vi "NI-DCPower Source DC Voltage.vi"() -> ()   [LabVIEW 2021]
doc: "Demonstrates how to use the DC Voltage Output Function to force an output voltage. This example initializes a session, configures the Output Function, Sense, Autorange, Voltage Level and Current Limit, initiates generation, waits for a specified delay, and measures the voltage and current output. This example uses Single Point source mode."
uses:
  <instrlib>/niDCPower/nidcpower.llb/niDCPower Source Mode.ctl
  <instrlib>/niDCPower/nidcpower.llb/niDCPower Wait For Event - Event.ctl
  <instrlib>/niDCPower/nidcpower.llb/niDCPower Output Function.ctl
  <instrlib>/niDigital/niDigital.llb/niDigital Selected Function.ctl
  <instrlib>/niDigital/niDigital.llb/niDigital Burst Pattern (Pass Fail).vi
  <instrlib>/niDigital/niDigital.llb/niDigital Get Site Results Site Numbers.vi
panel:
  out "Pass?":bool[](array[boolean])
  out "Site":string[](array[string])
  in  "Digital":refnum<k15>="PXI1Slot2,PXI1Slot3" caption="resource name"
  in  "error in":errorcluster
  out "error out":errorcluster
  in  "Source Delay (Sec)":dbl=0.1 format="%.3p"
  out "Voltage Measurement":dbl
  out "Current Measurement":dbl
  in  "Current Limit Range":dbl=0.01 format="%.3p"
  in  "Voltage Level Range":dbl=6.0 format="%.5p"
  in  "Current Limit":dbl=0.01 format="%.3p"
  in  "Voltage Level":dbl=2.0 format="%.5p"
  in  "Vin SMU Channel":string="0"
  in  "Vin SMU":refnum<k15>="Dev1"
  # "Overview: Demonstrates how to use the DC Voltage Output Function to force an output voltage.  \nThis example initializes a session; configures the Output Function, Voltage Level and Current Limit; \ninitiates generation; waits for a specified delay; and measures the voltage and current output. \nRequirements: NI-DCPower\nInstructions:\n1. Select the appropriate device in the Resource Name control.\n2. Configure the parameters of the DC Voltage signal you'd like to output.\n3. Run the VI."
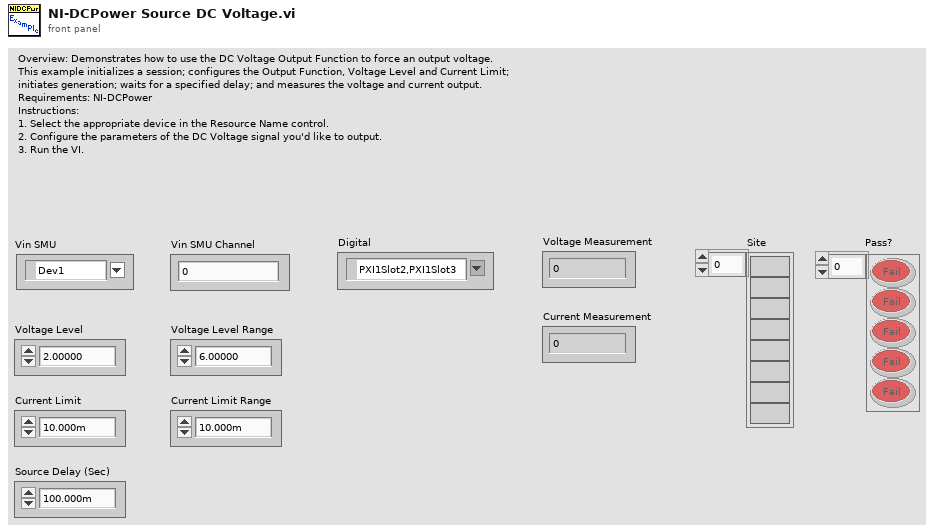
[diagram p1: front panel]
types:
  T1 = typedef "niDigital Selected Function.ctl" = i32
  T2 = typedef "niDCPower Output Function.ctl" = i32
  T3 = typedef "niDCPower Wait For Event - Event.ctl" = i32
  T4 = typedef "niDCPower Source Mode.ctl" = i32
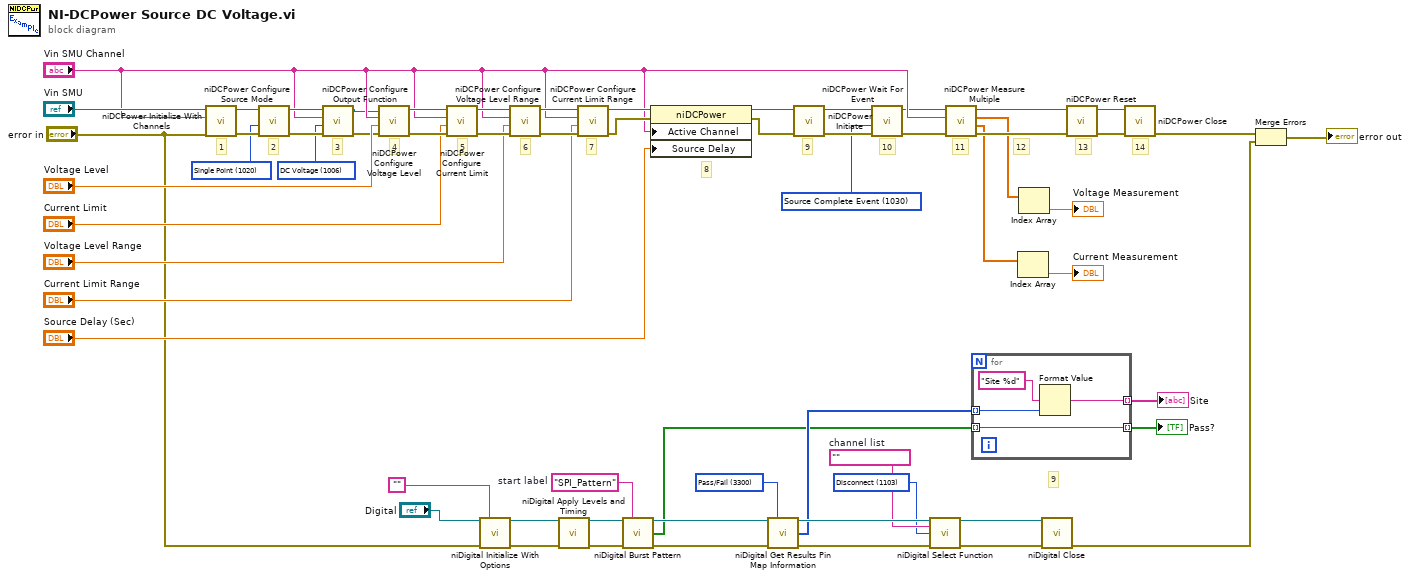
[diagram p0: block diagram]
diagram:
  w15 = ""  # channel list
  w14 = T1 1103 items=["Digital"=1100, "PPMU"=1101, "Off"=1102, "Disconnect"=1103] ("function")
  w9 = "SPI_Pattern"  # start label
  w13 = 3300 items=["Pass/Fail"=3300, "Capture Waveform"=3301] ("site result type")
  w29 = T2 1006 items=["DC Voltage"=1006, "DC Current"=1007, "Pulse Voltage"=1049, "Pulse Current"=1050] ("output function")
  w32 = T3 1030 items=["Source Complete Event"=1030, "Measure Complete Event"=1031, "Sequence Iteration Complete Event"=1032, "Sequence Engine Done Event"=1033] ("event")
  w51 = T4 1020 items=["Single Point"=1020, "Sequence"=1021] ("source mode")
  # "9"
  # "14"
  # "9"
  # "11"
  # "10"
  # "7"
  # "6"
  # "2"
  # "3"
  # "12"
  # "13"
  # "8"
  # "5"
  # "4"
  # "1"
  n1 = call <instrlib>:"niDCPower Initialize With Channels.vi"("error in (no error)"="error in", "channels"="Vin SMU Channel", "resource name"="Vin SMU") -> ("error out"=w55:errorcluster, "instrument handle out"=w54:refnum<k15>)  [unwired: 2 in, 5 out]
  n2 = call <instrlib>:"niDCPower Configure Source Mode.vi"("error in (no error)"=w55, "source mode"=w51, "instrument handle"=w54) -> ("error out"=w53:errorcluster, "instrument handle out"=w52:refnum<k15>)  [unwired: 7 out]
  n3 = call <instrlib>:"niDCPower Configure Output Function.vi"("error in (no error)"=w53, "output function"=w29, "channel name"="Vin SMU Channel", "instrument handle"=w52) -> ("error out"=w30:errorcluster, "instrument handle out"=w31:refnum<k15>)  [unwired: 6 out]
  n4 = call <instrlib>:"niDCPower Configure Voltage Level.vi"("error in (no error)"=w30, "voltage level"="Voltage Level", "channel name"="Vin SMU Channel", "instrument handle"=w31) -> ("error out"=w60:errorcluster, "instrument handle out"=w61:refnum<k15>)  [unwired: 6 out]
  n5 = call <instrlib>:"niDCPower Configure Current Limit.vi"("error in (no error)"=w60, "current limit"="Current Limit", "channel name"="Vin SMU Channel", "instrument handle"=w61) -> ("error out"=w50:errorcluster, "instrument handle out"=w49:refnum<k15>)  [unwired: 1 in, 5 out]
  n6 = call <instrlib>:"niDigital Initialize With Options.vi"("resource name"="Digital", "option string"="", "error in"="error in") -> ("instrument handle"=w22:refnum<k15>, "error out"=w23:errorcluster)  [unwired: 11 in]
  n7 = call <instrlib>:"niDCPower Configure Voltage Level Range.vi"("error in (no error)"=w50, "voltage level range"="Voltage Level Range", "channel name"="Vin SMU Channel", "instrument handle"=w49) -> ("error out"=w48:errorcluster, "instrument handle out"=w47:refnum<k15>)  [unwired: 6 out]
  n8 = call <instrlib>:"niDigital Apply Levels and Timing.vi"("instrument handle"=w22, "error in"=w23) -> ("instrument handle out"=w8:refnum<k15>, "error out"=w7:errorcluster)  [unwired: 12 in]
  n9 = call <instrlib>:"niDCPower Configure Current Limit Range.vi"("error in (no error)"=w48, "current limit range"="Current Limit Range", "channel name"="Vin SMU Channel", "instrument handle"=w47) -> ("error out"=w39:errorcluster, "instrument handle out"=w42:refnum<k15>)  [unwired: 6 out]
  n10 = call-poly <instrlib>:"niDigital Burst Pattern.vi"("instrument handle"=w8, "start label"=w9, "error in"=w7) -> ("instrument handle out"=w10:refnum<k15>, "pass"=w6:bool[], "error out"=w11:errorcluster)  [unwired: 10 in]
  n11 = property class="niDCPower"(reference=w42, error in=w39, "Active Channel"="Vin SMU Channel", "Source Delay"="Source Delay (Sec)") -> (reference out=w41:refnum<k15>, error out=w40:errorcluster)
  n12 = call-poly <instrlib>:"niDigital Get Results Pin Map Information.vi"("instrument handle"=w10, "site result type"=w13, "error in"=w11) -> ("instrument handle out"=w16:refnum<k15>, "site numbers"=w12:i32[], "error out"=w17:errorcluster)  [unwired: 10 in]
  n13 = call <instrlib>:"niDCPower Initiate.vi"("error in (no error)"=w40, "instrument handle"=w41) -> ("error out"=w34:errorcluster, "instrument handle out"=w36:refnum<k15>)  [unwired: 2 in, 6 out]
  n14 = call <instrlib>:"niDCPower Wait For Event.vi"("error in (no error)"=w34, "event"=w32, "instrument handle"=w36) -> ("error out"=w33:errorcluster, "instrument handle out"=w35:refnum<k15>)  [unwired: 1 in, 6 out]
  n15 = call <instrlib>:"niDigital Select Function.vi"("instrument handle"=w16, "channel list"=w15, "function"=w14, "error in"=w17) -> ("instrument handle out"=w19:refnum<k15>, "error out"=w18:errorcluster)  [unwired: 10 in]
  n16 = call <instrlib>:"niDCPower Measure Multiple.vi"("error in (no error)"=w33, "channel name"="Vin SMU Channel", "instrument handle"=w35) -> ("error out"=w43:errorcluster, "current measurements"=w27:dbl[], "voltage measurements"=w25:dbl[], "instrument handle out"=w44:refnum<k15>)  [unwired: 5 out]
  n17 = for {
    tunnel: w6 -> [w63] mode=indexing
    tunnel: w12 -> [w65] mode=indexing
    tunnel: [w64] -> w2 mode=indexing
    tunnel: [w63] -> w1 mode=indexing
    n18 = Format Value(format string="Site %d", value (0)=w65) -> (output string=w64:string)  [unwired: 1 in]
  }
  "Site" <- w2
  "Pass?" <- w1
  n19 = Index Array(array=w27) -> (element=→"Current Measurement":dbl)  [unwired: 1 in]
  n20 = Index Array(array=w25) -> (element=→"Voltage Measurement":dbl)  [unwired: 1 in]
  n21 = call <instrlib>:"niDigital Close.vi"("instrument handle"=w19, "error in"=w18) -> ("error out"=w4:errorcluster)  [unwired: 13 in]
  n22 = call <instrlib>:"niDCPower Reset.vi"("error in (no error)"=w43, "instrument handle"=w44) -> ("error out"=w57:errorcluster, "instrument handle out"=w58:refnum<k15>)  [unwired: 2 in, 6 out]
  n23 = call <instrlib>:"niDCPower Close.vi"("error in (no error)"=w57, "instrument handle"=w58) -> ("error out"=w28:errorcluster)  [unwired: 9 out]
  n24 = Merge Errors(w28, w4) -> (→"error out":errorcluster)
